vi "testVI.vi"() -> ()   [LabVIEW 2023]
panel:
  out "Waveform Chart":dbl[][](graph)
  out "y":dbl[](array[numeric]) format="%.4f"
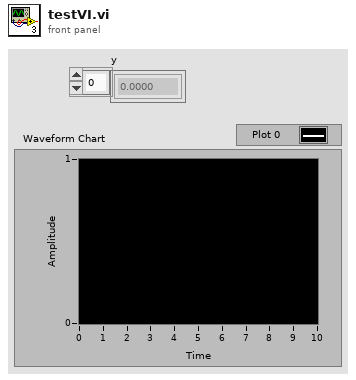
[diagram p1: front panel]
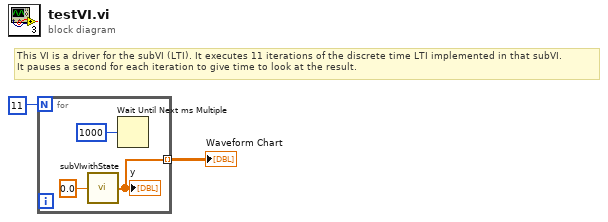
[diagram p0: block diagram]
diagram:
  # "This VI is a driver for the subVI (LTI). It executes 11 iterations of the discrete time LTI implemented in that subVI.\nIt pauses a second for each iteration to give time to look at the result."
  n1 = for {
    N: 11 -> [_]
    tunnel: [w3] -> w1 mode=indexing
    n2 = call "subVIwithState.vi"("u"=0.0) -> ("y"=w3:dbl[])
    "y" <- w3
    n3 = Wait Until Next ms Multiple(millisecond multiple=u32 1000) -> ()  [unwired: 1 out]
  }
  "Waveform Chart" <- w1
